vi "NI Minimize Window.vi"(8 "error in (no error)":errorcluster, 11 "window name  (\"\")":string) -> (0 "error out":errorcluster)   [LabVIEW 2018]
doc: "This function will minimize the window named in the window name input, or identified by the window refnum. If an invalid window refnum is passed in, then the function will use the window name to get a window window refnum. If the window cannot be found, an error will be returned."
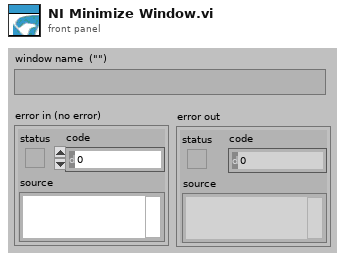
[diagram p1: front panel]
types:
  T1 = enum8{"Maximize Window", "Minimize Window", "Show Task List", "Start Screen Saver", "Quit Application"}
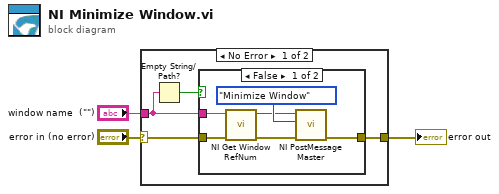
[diagram p0: block diagram]
diagram:
  n1 = case shown="No Error" "error in (no error)" {
    selector: "error in (no error)" -> [w6 w15]
    tunnel: [w7 w15] -> w2
    tunnel: "window name  (\"\")" -> [w4 _]
    frame No Error {
      n2 = Empty String/Path?(string/path=w4) -> (empty?=w5:bool)
      n3 = case shown="False" w5 {
        tunnel: [w13 w14] -> w7
        tunnel: w4 -> [w10 _]
        tunnel: w6 -> [w11 w14]
        frame False {
          n4 = call "NI Get Window RefNum.vi"("error in (no error)"=w11, "window name (\"\")"=w10) -> ("error out"=w8:errorcluster, "window refnum (NaWR)"=w9:refnum<k1>)  [unwired: 8 in]
          n5 = call "NI PostMessage Master.vi"("error in (no error)"=w8, "function"=T1."Minimize Window", "window refnum"=w9) -> ("error out"=w13:errorcluster)  [unwired: 8 in]
        }
        frame True {
        }
      }
    }
    frame Error {
    }
  }
  "error out" <- w2
